vi "Force and position waveforms.vi"(0 "Input waveforms":waveform(dbl)[](array[waveform]), 1 "Forces  (pN)":dbl[][](array[numeric]), 2 "Deflections (nm)":dbl[][](array[numeric]), 3 "Mean Trap Positions (nm)":T1={"T1 X"=3248.000000000121, "T2 X"=6090.0, "T3 X"=4120.979470198669, "T3 Y"=2049.2494705038607} {"T3 Y" format="%#_6f"; "T3 X" format="%#_6f"; "T2 X" format="%#_6f"; "T1 X" format="%#_6f"}) -> (4 "1D data":waveform(dbl)[](array[waveform]), 5 "Absolute Positions":waveform(dbl)[](array[waveform]), 6 "Forces":waveform(dbl)[](array[waveform]), 7 "Deflections":waveform(dbl)[](array[waveform]), 8 "Raw Data":waveform(dbl)[](array[waveform]))   [LabVIEW 2014]
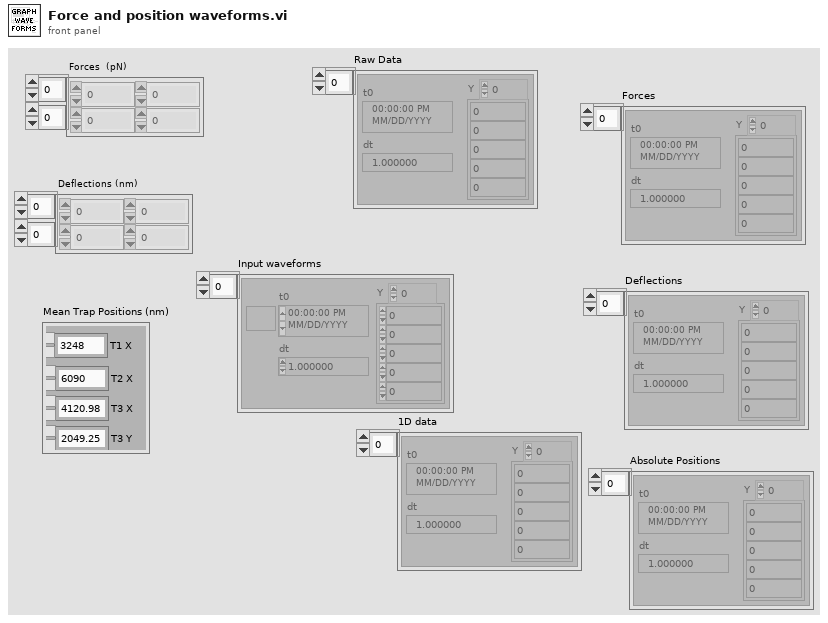
[diagram p1: front panel]
types:
  T1 = cluster{"T1 X":dbl, "T2 X":dbl, "T3 X":dbl, "T3 Y":dbl}
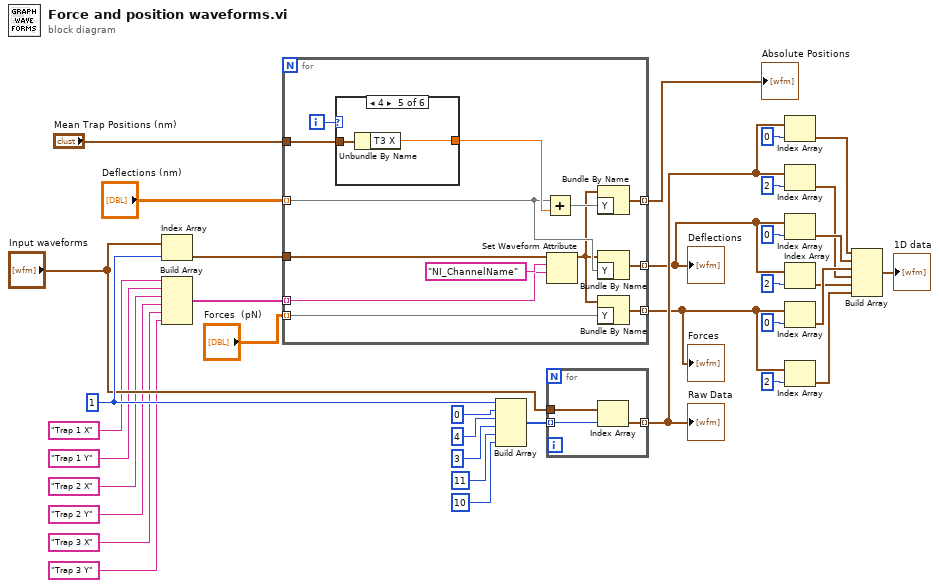
[diagram p0: block diagram]
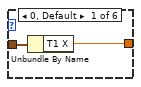
[diagram p2: hidden frame]
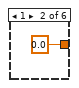
[diagram p3: hidden frame]
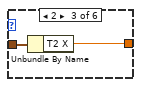
[diagram p4: hidden frame]
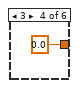
[diagram p5: hidden frame]
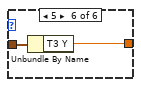
[diagram p6: hidden frame]
diagram:
  w26 = 1
  n1 = Index Array(array="Input waveforms", index=w26) -> (element=w32:waveform(dbl))
  n2 = Build Array("Trap 1 X", "Trap 1 Y", "Trap 2 X", "Trap 2 Y", "Trap 3 X", "Trap 3 Y") -> (w1:string[])
  n3 = for {
    tunnel: w32 -> [w40]
    tunnel: "Forces  (pN)" -> [w49] mode=indexing
    tunnel: "Deflections (nm)" -> [w45] mode=indexing
    tunnel: "Mean Trap Positions (nm)" -> [w47]
    tunnel: [w43] -> w16 mode=indexing
    tunnel: [w42] -> w15 mode=indexing
    tunnel: [w41] -> w33 mode=indexing
    tunnel: w1 -> [w37] mode=indexing
    i -> [w48]
    n4 = case shown="4" w48 {
      tunnel: w47 -> [w51 _ w54 _ w57 w59]
      tunnel: [w50 0.0 w53 0.0 w56 w58] -> w46
      frame 0, Default {
        n5 = Unbundle By Name(w51) -> ("T1 X"=w50:dbl)
      }
      frame 1 {
      }
      frame 2 {
        n6 = Unbundle By Name(w54) -> ("T2 X"=w53:dbl)
      }
      frame 3 {
      }
      frame 4 {
        n7 = Unbundle By Name(w57) -> ("T3 X"=w56:dbl)
      }
      frame 5 {
        n8 = Unbundle By Name(w59) -> ("T3 Y"=w58:dbl)
      }
    }
    n9 = Add(x=w45, y=w46) -> (x+y=w44:dbl[])
    n10 = Set Waveform Attribute(5:w37, 6:"NI_ChannelName", 7:w40) -> (3:w39:waveform(dbl))  [unwired: 1 in, 2 out]
    n11 = Bundle By Name(cluster=w39, "Y"=w44) -> (w41:waveform(dbl))
    n12 = Bundle By Name(cluster=w39, "Y"=w45) -> (w42:waveform(dbl))
    n13 = Bundle By Name(cluster=w39, "Y"=w49) -> (w43:waveform(dbl))
  }
  "Forces" <- w16
  "Deflections" <- w15
  "Absolute Positions" <- w33
  n14 = Build Array(w26, 0, 4, 3, 11, 10) -> (w25:i32[])
  n15 = for {
    tunnel: w25 -> [w62] mode=indexing
    tunnel: "Input waveforms" -> [w61]
    tunnel: [w60] -> w17 mode=indexing
    n16 = Index Array(array=w61, index=w62) -> (element=w60:waveform(dbl))
  }
  "Raw Data" <- w17
  n17 = Index Array(array=w17, index=0) -> (element=w14:waveform(dbl))
  n18 = Index Array(array=w17, index=2) -> (element=w11:waveform(dbl))
  n19 = Index Array(array=w15, index=0) -> (element=w13:waveform(dbl))
  n20 = Index Array(array=w15, index=2) -> (element=w10:waveform(dbl))
  n21 = Index Array(array=w16, index=0) -> (element=w12:waveform(dbl))
  n22 = Index Array(array=w16, index=2) -> (element=w9:waveform(dbl))
  n23 = Build Array(w14, w13, w12, w11, w10, w9) -> (→"1D data":waveform(dbl)[])
